vi "Status Message.vi"(7 "Error In":errorcluster, 8 "Start/End":bool, 9 "Step #":i32, 10 "Message":string) -> (0 "Error Out":errorcluster, 1 "Status":variant)   [LabVIEW 2018]
uses:
  Controls/Status Message.ctl
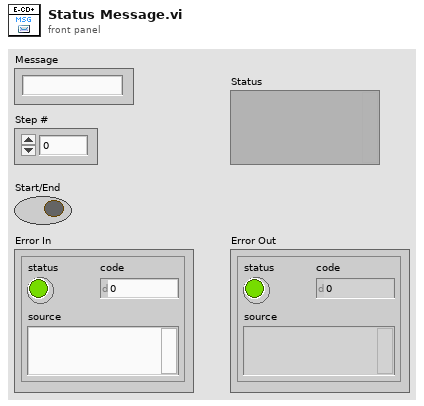
[diagram p1: front panel]
types:
  T1 = typedef "Status Message.ctl" = cluster{"Message":string, "Step #":i32, "Start/End":bool}
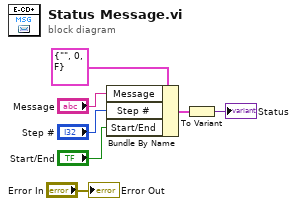
[diagram p0: block diagram]
diagram:
  n1 = Bundle By Name(cluster=T1 {"Message"="", "Step #"=0, "Start/End"=FALSE} ("Status Message"), "Message"="Message", "Step #"="Step #", "Start/End"="Start/End") -> (w7:T1)
  n2 = To Variant(anything=w7) -> (Variant=→"Status":variant)
  "Error Out" <- "Error In"
